vi "Drive Controller.vi"(8 "error in":errorcluster) -> ()   [LabVIEW 2020]
doc: "This VI executes continuously carrying out the current operation and responding to updates or new operation requests. It will often contain the timing or control code that is difficult to place directly in TeleOp. This VI generally opens all sensors and motors and isolates the rest of the robot code from knowing implementation details of how the operations are carried out."
uses:
  <vilib>/Rock Robotics/WPI/Framework/Completion Status.ctl
  Drive Setpoints.ctl
  Drive Operations.ctl
  <vilib>/Rock Robotics/WPI/ThirdParty/Phoenix-LabVIEW/Motor Controller/Controls/CTRE_Phoenix_MotorControl_ControlMode.ctl
panel:
  in  "Interactive Values":T1
  in  "Buttons":cluster{"Execute Cmd":bool, "Abort Cmd":bool}
  out "Command Timing":cluster{"Start Time (ms)":u32, "Iterations":i32}
  out "Status":T3
  out "Setpoints":T4(graph)
  out "Current\nCmd":string
  # "Tip: The graph shows the motor setpoints. It may also be helpful to observe inputs and sensor values.\nYou may also want to display tuning or debugging controls."
  # "Interactive Command: You may fill in the settings for a command\nand schedule it with the Execute button. You can observe and abort\nany command while fine tuning the code for the controller."
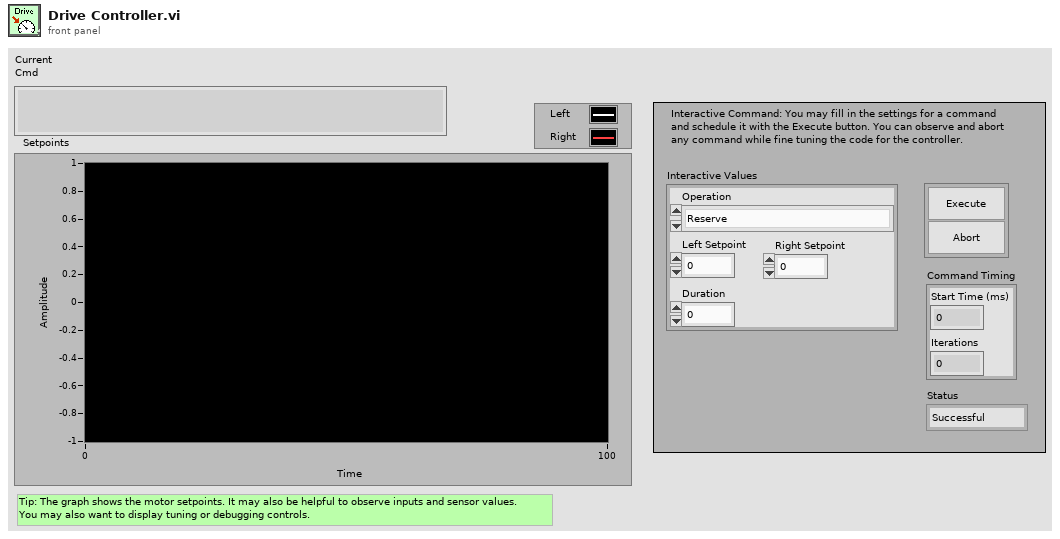
[diagram p1: front panel]
types:
  T1 = typedef "Drive Setpoints.ctl" = cluster{"Operation":T2, "Left Setpoint":dbl, "Right Setpoint":dbl, "Duration":dbl}
  T2 = typedef "Drive Operations.ctl" = enum16{"Reserve", "Read Current", "Immediate", "Drive for Time", "Drive for Distance"}
  T3 = typedef "Completion Status.ctl" = enum16{"Successful", "Aborted", "Incomplete"}
  T4 = cluster{"Left Setpoint":dbl, "Right Setpoint":dbl}
  T5 = typedef "WPI_MotorControlDeviceRef.ctl" = cluster{"DeviceStatus":errorcluster, "Type":T6, "PWM":cluster{"PWM Channel":T7, "DeadBand":T8}, "CAN":cluster{"Device Number":u8, "SetOutput VI Ref":variant, "GetOutput VI Ref":variant, "Enable VI Ref":variant, "Disable VI Ref":variant, "Data":variant}, "Invert":bool, "DIO PWM":cluster{"PWM \"Enable\" Channel":T7, "DIOChannel":T9, "PWM Rate":dbl}}
  T6 = typedef "WPI_MotorControlType.ctl" = enum16{"PWM", "CAN", "DIO PWM"}
  T7 = typedef "FPGA_DIOPWMChannel.ctl" = enum8{"PWM 0", "PWM 1", "PWM 2", "PWM 3", "PWM 4", "PWM 5", "PWM 6", "PWM 7", "PWM 8", "PWM 9", "PWM MXP 0", "PWM MXP 1", "PWM MXP 2", "PWM MXP 3", "PWM MXP 4", "PWM MXP 5", "PWM MXP 6", "PWM MXP 7", "PWM MXP 8", "PWM MXP 9", "Invalid"}
  T8 = typedef "WPI_PWMDeadband.ctl" = cluster{"Name":string, "maxPositivePwm":i32, "minPositivePwm":i32, "centerPwm":i32, "maxNegativePwm":i32, "minNegativePwm":i32, "angularRange":u16}
  T9 = typedef "FPGA_DIOChannel.ctl" = enum8{"DIO 0", "DIO 1", "DIO 2", "DIO 3", "DIO 4", "DIO 5", "DIO 6", "DIO 7", "DIO 8", "DIO 9", "DIO MXP 0", "DIO MXP 1", "DIO MXP 2", "DIO MXP 3", "DIO MXP 4", "DIO MXP 5", "DIO MXP 6", "DIO MXP 7", "DIO MXP 8", "DIO MXP 9", "DIO MXP 10", "DIO MXP 11", "DIO MXP 12", "DIO MXP 13", "DIO MXP 14", "DIO MXP 15", "SPI Port CS1", "SPI Port CS2", "SPI Port CS3", "SPI Port MISO", "SPI Port MOSI", "Invalid"}
  T10 = typedef "Command Status Info.ctl" = cluster{"Name":string, "Status":T3, "notifier out":T11}
  T11 = typedef "Completion Notifier.ctl" = refnum<notifier>
  T12 = cluster{"SubSystem Data":T1, cluster{"Start Time (ms)":u32, "Iterations":i32}, cluster{"Command Info":T10, "Description":string, "Default Command":T1, "queue out":refnum<queue>, "Subsystem Name":string}}
  T13 = typedef "CTRE_Phoenix_MotorControl_ControlMode.ctl" = u16
  T14 = cluster{"SubSystem Data":T1, cluster{"Start Time (ms)":u32, "Iterations":i32}, "Default Command Arguments":cluster{"Command Info":T10, "Description":string, "Default Command":T1, "queue out":refnum<queue>, "Subsystem Name":string}}
  T15 = cluster{"Don't move motors while reserved":dbl, "Don't move motors while reserved":dbl}
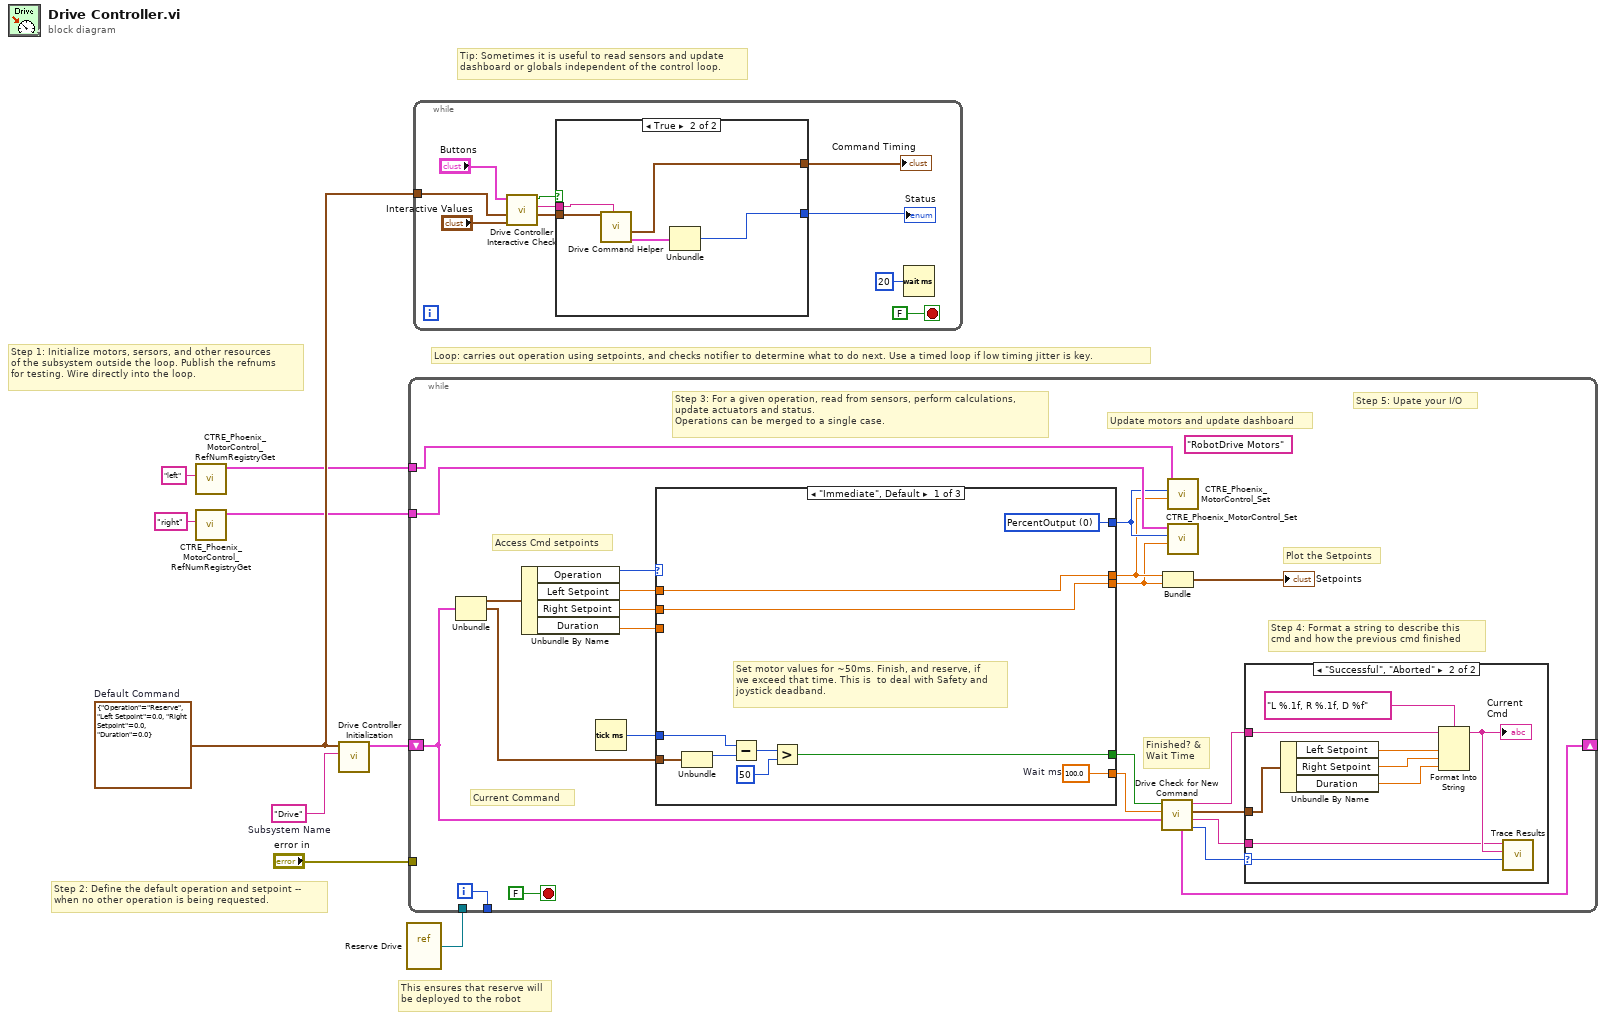
[diagram p0: block diagram]
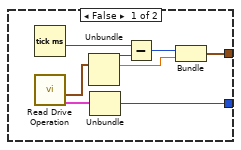
[diagram p2: hidden frame]
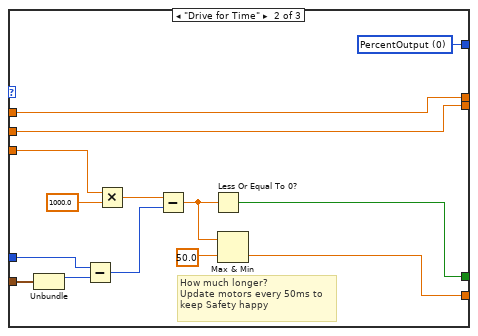
[diagram p4: hidden frame]
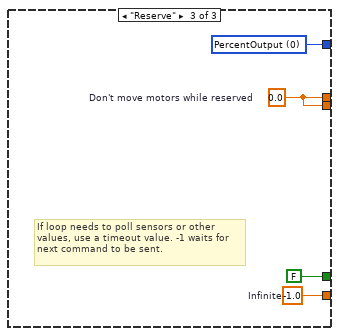
[diagram p5: hidden frame]
diagram:
  w5 = T1 {"Operation"=enum."Reserve", "Left Setpoint"=0.0, "Right Setpoint"=0.0, "Duration"=0.0}  # Default Command
  w9 = "Drive"  # Subsystem Name
  # "This ensures that reserve will\nbe deployed to the robot"
  # "Tip: Sometimes it is useful to read sensors and update\ndashboard or globals independent of the control loop."
  # "Step 2: Define the default operation and setpoint --\nwhen no other operation is being requested."
  # "Step 1: Initialize motors, sersors, and other resources\nof the subsystem outside the loop. Publish the refnums\nfor testing. Wire directly into the loop."
  # "Loop: carries out operation using setpoints, and checks notifier to determine what to do next. Use a timed loop if low timing jitter is key."
  n1 = call <vilib>:"CTRE_Phoenix_MotorControl_RefNumRegistryGet.vi"("refnum name"="left") -> ("PhoenixMotorControlDevRef"=w2:T5)  [unwired: 9 in, 1 out]
  n2 = call <vilib>:"CTRE_Phoenix_MotorControl_RefNumRegistryGet.vi"("refnum name"="right") -> ("PhoenixMotorControlDevRef"=w1:T5)  [unwired: 9 in, 1 out]
  n3 = call "Drive Controller Initialization.vi"("Subsystem Name"=w9, "Default Command"=w5) -> ("Current Command"=w7:T12)  [unwired: 9 in]
  n4 = vi-ref "Reserve Drive.vi"() -> (w6:refnum<vi>)
  n5 = while {
    shift-right: [w22] -> _
    shift-left: w7 -> [w15]
    tunnel: [w31] -> _
    tunnel: "error in" -> [_]
    tunnel: w6 -> [_]
    tunnel: w2 -> [w14]
    tunnel: w1 -> [w13]
    i -> [w31]
    stop <- FALSE stop-if-true
    (unwired) "RobotDrive Motors" ("Name")
    # "Step 5: Upate your I/O"
    # "Step 4: Format a string to describe this\ncmd and how the previous cmd finished"
    # "Current Command"
    # "Update motors and update dashboard"
    # "Plot the Setpoints"
    # "Access Cmd setpoints"
    # "Finished? &\nWait Time"
    # "Step 3: For a given operation, read from sensors, perform calculations,\nupdate actuators and status.\nOperations can be merged to a single case."
    n6 = Unbundle(w15) -> ("SubSystem Data"=w29:T1, w16:cluster{"Start Time (ms)":u32, "Iterations":i32})  [unwired: 1 out]
    n7 = Unbundle By Name(w29) -> ("Operation"=w28:T2, "Left Setpoint"=w27:dbl, "Right Setpoint"=w26:dbl, "Duration"=w25:dbl)
    n8 = Tick Count (ms)() -> (millisecond timer value=w24:u32)
    n9 = case shown="\"Immediate\", Default" w28 {
      tunnel: [w51 w53 w69] -> w21
      tunnel: [w44 w60 FALSE ("ignore previous (F)")] -> w20
      tunnel: w16 -> [w43 w62 _]
      tunnel: [w50 w59 w66] -> w11
      tunnel: [w49 w58 w66] -> w10
      tunnel: w27 -> [w50 w59 _]
      tunnel: w26 -> [w49 w58 _]
      tunnel: w25 -> [_ w57 _]
      tunnel: w24 -> [w45 w56 _]
      tunnel: [w42 w52 w67] -> w12
      frame "Immediate", Default {
        w42 = T13 0 items=["PercentOutput"=0, "Position"=1, "Velocity"=2, "Current"=3, "Follower"=5, "MotionProfile"=6, "MotionMagic"=7, "MotionProfileArc"=10, "Disabled"=15] ("Control Mode")
        w51 = 100.0  # Wait ms
        # "Set motor values for ~50ms. Finish, and reserve, if\nwe exceed that time. This is  to deal with Safety and\njoystick deadband."
        n10 = Unbundle(w43) -> ("Start Time (ms)"=w46:u32)  [unwired: 1 out]
        n11 = Subtract(x=w45, y=w46) -> (x-y=w47:u32)
        n12 = Greater?(x=w47, y=u8 50 ("Left Motor")) -> (0:w44:bool)
      }
      frame "Drive for Time" {
        w52 = T13 0 items=["PercentOutput"=0, "Position"=1, "Velocity"=2, "Current"=3, "Follower"=5, "MotionProfile"=6, "MotionMagic"=7, "MotionProfileArc"=10, "Disabled"=15] ("Control Mode")
        # "How much longer?\nUpdate motors every 50ms to\nkeep Safety happy"
        n13 = Unbundle(w62) -> ("Start Time (ms)"=w61:u32)  [unwired: 1 out]
        n14 = Subtract(x=w56, y=w61) -> (x-y=w65:u32)
        n15 = Multiply(x=w57, y=1000.0) -> (x*y=w64:dbl)
        n16 = Subtract(x=w64, y=w65) -> (x-y=w55:dbl)
        n17 = Less Or Equal To 0?(x=w55) -> (x <= 0?=w60:bool)
        n18 = Max & Min(x=w55, y=50.0) -> (min(x,y)=w53:dbl)  [unwired: 1 out]
      }
      frame "Reserve" {
        w67 = T13 0 items=["PercentOutput"=0, "Position"=1, "Velocity"=2, "Current"=3, "Follower"=5, "MotionProfile"=6, "MotionMagic"=7, "MotionProfileArc"=10, "Disabled"=15] ("Control Mode")
        w66 = 0.0  # Don't move motors while reserved
        w69 = -1.0  # Infinite
        # "If loop needs to poll sensors or other\nvalues, use a timeout value. -1 waits for\nnext command to be sent."
      }
    }
    n19 = call "Drive Check for New Command.vi"("input cluster"=w15, "Wait time (ms)"=w21, "Finished?"=w20) -> ("Completion"=w23:T3, "Subsystem Name"=w17:string, "Current Command"=w18:T1, "Initial Trace String"=w19:string, "Next Command"=w22:T14)  [unwired: 4 in]
    n20 = Bundle("Don't move motors while reserved"=w11, "Don't move motors while reserved"=w10) -> (→"Setpoints":T15)  [unwired: 1 in]
    n21 = call <vilib>:"CTRE_Phoenix_MotorControl_Set.vi"("Output"=w11, "Control Mode"=w12, "PhoenixMotorControlDevRef"=w14) -> ()  [unwired: 7 in, 2 out]
    n22 = call <vilib>:"CTRE_Phoenix_MotorControl_Set.vi"("Output"=w10, "Control Mode"=w12, "PhoenixMotorControlDevRef"=w13) -> ()  [unwired: 7 in, 2 out]
    n23 = case shown="\"Successful\", \"Aborted\"" w23 {
      selector: w23 -> [_ w41]
      tunnel: w19 -> [_ w36]
      tunnel: w18 -> [_ w37]
      tunnel: w17 -> [_ w33]
      frame "Incomplete", Default {
        # "Continuing current command"
      }
      frame "Successful", "Aborted" {
        # "Report and setup for next command"
        n24 = Unbundle By Name(w37) -> ("Left Setpoint"=w39:dbl, "Right Setpoint"=w40:dbl, "Duration"=w34:dbl)
        n25 = Format Into String(format string="L %.1f, R %.1f, D %f", initial string=w36, w39, w40, w34) -> (resulting string=w35:string)  [unwired: 1 in, 1 out]
        "Current\nCmd" <- w35
        n26 = call <vilib>:"Trace Results.vi"("Status of previous command"=w41, "Description"=w35, "Subsystem"=w33) -> ()  [unwired: 9 in]
      }
    }
  }
  n27 = while {
    tunnel: w5 -> [w71]
    stop <- FALSE stop-if-true
    n28 = call "Drive Controller Interactive Check.vi"("Interactive Command In"="Interactive Values", "Default Command"=w71, "Buttons"="Buttons") -> ("Interactive Command Out"=w73:T1, "Trace String"=w74:string, "Schedule"=w75:bool)  [unwired: 6 in]
    n29 = case shown="True" w75 {
      tunnel: [w84 w92] -> w76
      tunnel: [w83 w88] -> w77
      tunnel: w74 -> [_ w90]
      tunnel: w73 -> [_ w89]
      frame False {
        n30 = Tick Count (ms)() -> (millisecond timer value=w87:u32)
        n31 = call "Read Drive Operation.vi"() -> ("Command Info"=w81:T10, "SubSystem Data"=w80:T1)  [unwired: 9 in, 1 out]
        n32 = Unbundle(w80) -> ("Operation"=w85:T2, "Left Setpoint"=w82:dbl)  [unwired: 2 out]
        n33 = Unbundle(w81) -> ("Status"=w84:T3)  [unwired: 2 out]
        n34 = Subtract(x=w87, y=w85) -> (x-y=w86:u32)
        n35 = Bundle(w86, "Left Setpoint"=w82) -> (w83:cluster{u32, "Left Setpoint":dbl})  [unwired: 1 in]
      }
      frame True {
        n36 = call "Drive Command Helper.vi"("Description"=w90, "SubSystem Data"=w89) -> ("Command Info Out"=w91:T10, "Command Timing"=w88:cluster{"Start Time (ms)":u32, "Iterations":i32})  [unwired: 7 in, 1 out]
        n37 = Unbundle(w91) -> ("Status"=w92:T3)  [unwired: 2 out]
      }
    }
    "Status" <- w76
    "Command Timing" <- w77
    n38 = Wait (ms)(milliseconds to wait=u32 20) -> ()  [unwired: 1 out]
  }
